vi "GetHintBoolean.vi"(8 "No Error":errorcluster, 10 "Default Value":bool, 11 "Hint Name":T1) -> (0 "error out":errorcluster, 3 "Value":bool)   [LabVIEW 2026, in "SDL3.lvlib" / "Hints.lvlib"]
doc: "<B>Summary</B>\nGet the boolean value of a hint variable."
uses:
  Hints.lvlib
  HintName--combobox.ctl
  Lib/SDL3.dll
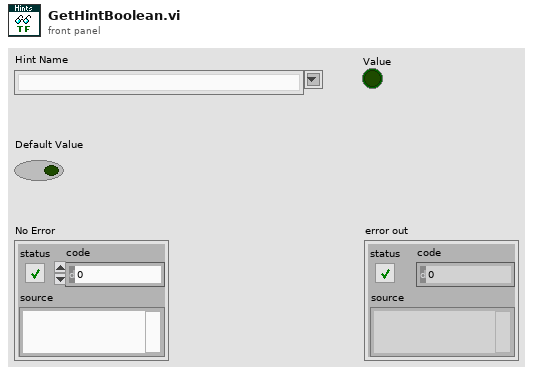
[diagram p1: front panel]
types:
  T1 = typedef "SDL3.lvlib/Hints.lvlib/HintName--combobox.ctl" = string
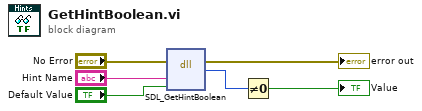
[diagram p0: block diagram]
diagram:
  n1 = dll-call lib="C:/Users/saukko/Dev/LV-SDL3/Sources/SDL3/Lib/SDL3.*" fn="SDL_GetHintBoolean"(error in="No Error", "name"="Hint Name", "default_value"="Default Value") -> (error out=→"error out":errorcluster, "return type"=w2:i32)  [unwired: 4 in, 1 out]
  n2 = Not Equal To 0?(x=w2) -> (x != 0?=→"Value":bool)
